vi "Error To Text.vi"(7 "Bench Module":T1=enum."4072", 8 "error in (no error)":errorcluster) -> (0 "error out":errorcluster, 3 "message":string=" INSTRUCTIONS:\r\rNormal Use:  When using subVIs that incorporate the error in/error out (or error I/O) structure, place this handler where you want to inform the user of an error, typically at the end of the I/O data path, as the last action of the program.  If the error in error? is ERROR, the handler creates a message describing the error and its source.  If the type of dialog = 1 (default), the message is displayed to the user, who can only acknowedge it.  If the type = 2, the user can acknowledge the message or abort execution; aborting a program with active I/O is not recommended.  If the type = 0, no message is displayed; this is used to process the error programmatically, and the error out cluster elements are wired to individual terminals for that reason.  \r\rOther Use:\n\r\nlocal testing.  To test the error code of a subVI or function that does not have the error I/O structure, you can wire its error code and a source string to the local error code and error source inputs.  If error in error? indicates no error and error code is not equal to 0, the local code and source are substituted for the error in values, and error? is set TRUE (ERROR).")   [LabVIEW 2026, in "PXI_Common.lvlib"]
uses:
  PXI_Common.lvlib
  Types/Enum/Bench Modules.ctl
  <vilib>/Utility/error.llb/DialogType.ctl
  Paths/Items/Custom Error Cfg Path.vi
  <vilib>/Utility/config.llb/Read Key (String).vi
  <vilib>/Utility/config.llb/NI_LVConfig.lvlib
  <vilib>/Utility/Data Type/NI_Data Type.lvlib
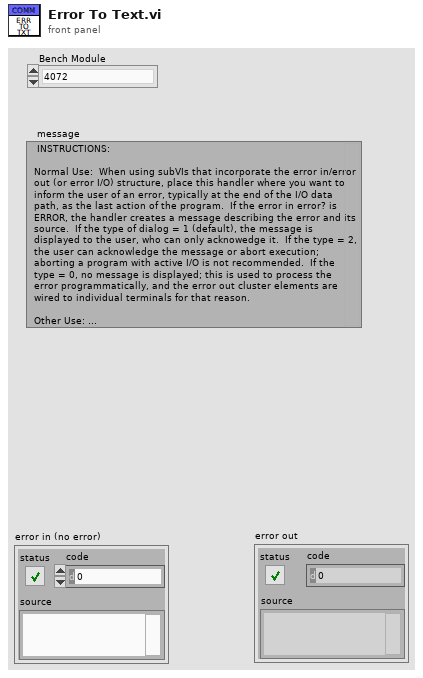
[diagram p1: front panel]
types:
  T1 = typedef "PXI_Common.lvlib/Bench Modules.ctl" = enum16{"Common", "4072", "6259", "6224", "4130", "8431"}
  T2 = typedef "DialogType.ctl" = u16
  T3 = typedef "NI_LVConfig.lvlib/Config Data RefNum.ctl" = refnum<k1>
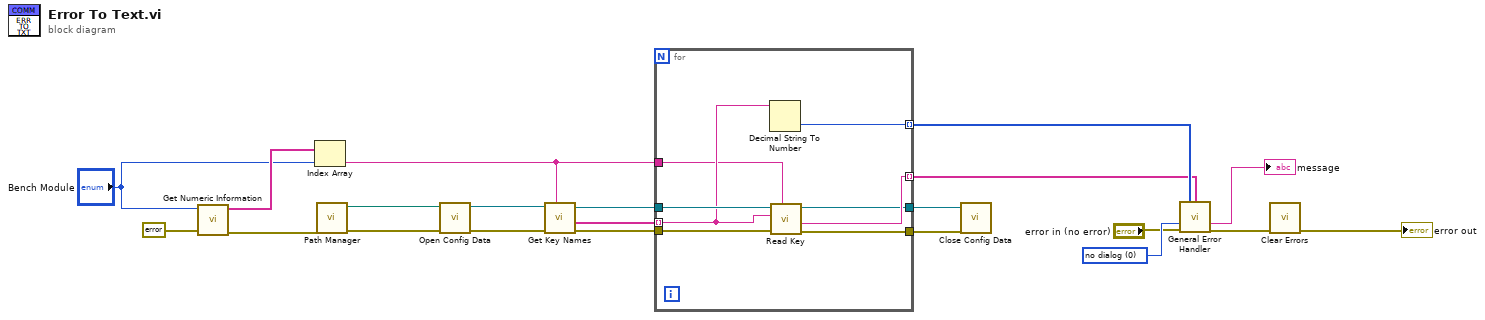
[diagram p0: block diagram]
diagram:
  w7 = T2 0 items=["no dialog", "OK message", "continue or stop message", "OK message + warnings", "continue/stop + warnings"] ("type of dialog (OK msg:1)")
  n1 = call <vilib>:"Get Numeric Information.vi"("error in (no error)"=errorcluster {"status"=FALSE, "code"=0, "source"=""} ("no error constant"), "variant"="Bench Module") -> ("error out"=w11:errorcluster, "enum names"=w10:string[])  [unwired: 6 in, 2 out]
  n2 = Index Array(array=w10, index="Bench Module") -> (element=w3:string)
  n3 = call-poly "Path Manager.vi"("error in (no error)"=w11) -> ("error out"=w20:errorcluster, "path"=w19:path)  [unwired: 9 in]
  n4 = call <vilib>:"Open Config Data.vi"("error in (no error)"=w20, "configuration file path"=w19) -> ("error out"=w18:errorcluster, "refnum"=w17:T3)  [unwired: 7 in, 1 out]
  n5 = call <vilib>:"Get Key Names.vi"("section"=w3, "error in (no error)"=w18, "refnum"=w17) -> ("error out"=w13:errorcluster, "key names"=w15:string[], "refnum out"=w14:T3)  [unwired: 5 in, 1 out]
  n6 = for {
    tunnel: [w29] -> w16
    tunnel: w15 -> [w24] mode=indexing
    tunnel: w14 -> [w28]
    tunnel: [w27] -> w4 mode=indexing
    tunnel: w13 -> [w26]
    tunnel: [w25] -> w12
    tunnel: [w22] -> w5 mode=indexing
    tunnel: w3 -> [w23]
    n7 = Decimal String To Number(string=w24) -> (number=w22:i32)  [unwired: 2 in, 1 out]
    n8 = call-poly <vilib>:"Read Key.vi"("section"=w23, "error in (no error)"=w26, "key"=w24, "refnum"=w28) -> ("error out"=w29:errorcluster, "value"=w27:string, "refnum out"=w25:T3)  [unwired: 4 in, 1 out]
  }
  n9 = call <vilib>:"Close Config Data.vi"("error in (no error)"=w16, "refnum"=w12) -> ()  [unwired: 8 in, 2 out]
  n10 = call <vilib>:"General Error Handler.vi"("[user-defined codes]"=w5, "[user-defined descriptions]"=w4, "type of dialog (OK msg:1)"=w7, "error in (no error)"="error in (no error)") -> ("message"=→"message":string, "error out"=w6:errorcluster)  [unwired: 7 in, 3 out]
  n11 = call <vilib>:"Clear Errors.vi"("error in (no error)"=w6) -> ("error out"=→"error out":errorcluster)  [unwired: 5 in, 1 out]
